vi "1D Array Find Closest Freq.vi"(8 "start index (0)":i32, 9 "Desired Element":dbl, 10 "Trace Data":dbl[](array[numeric]) format="%^.3e", 11 "Trace Freq":dbl[](array[numeric])) -> (2 "Close Trace Data":dbl, 3 "Closest Trace Freq":dbl)   [LabVIEW 2015]
panel:
  out "closest index":i32
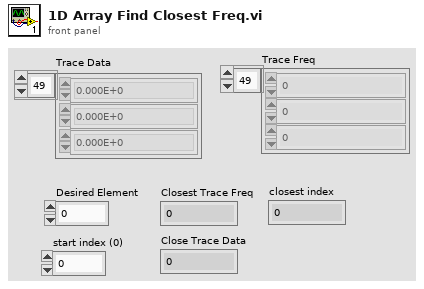
[diagram p1: front panel]
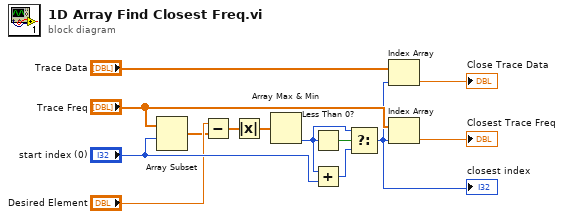
[diagram p0: block diagram]
diagram:
  n1 = Array Subset(array="Trace Freq", index="start index (0)") -> (w5:dbl[])  [unwired: 1 in]
  n2 = Subtract(x="Desired Element", y=w5) -> (x-y=w13:dbl[])
  n3 = Absolute Value(x=w13) -> (abs(x)=w10:dbl[])
  n4 = Array Max & Min(array=w10) -> (min index (indices)=w8:i32)  [unwired: 3 out]
  n5 = Less Than 0?(x=w8) -> (x < 0?=w9:bool)
  n6 = Add(x=w8, y="start index (0)") -> (x+y=w7:i32)
  n7 = Select(t=w8, s=w9, f=w7) -> (s? t:f=w1:i32)
  "closest index" <- w1
  n8 = Index Array(array="Trace Data", index=w1) -> (element=→"Close Trace Data":dbl)
  n9 = Index Array(array="Trace Freq", index=w1) -> (element=→"Closest Trace Freq":dbl)
